vi "BlueM_Excel-gain.vi"() -> ()   [LabVIEW 2018]
panel:
  out "PID gain schedule":T1(array[cluster])=[{"PID gains"={"proportional gain (Kc)"=1.0, "integral time (Ti, min)"=0.01, "derivative time (Td, min)"=0.0}, "max value"=100.0}] {"max value" format="%.2f"; "PID gains"."derivative time (Td, min)" format="%.3f"; "PID gains"."integral time (Ti, min)" format="%.3f"; "PID gains"."proportional gain (Kc)" format="%.3f"}
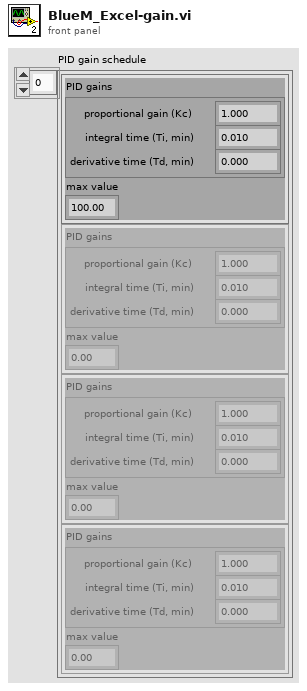
[diagram p1: front panel]
types:
  T1 = cluster{"PID gains":cluster{"proportional gain (Kc)":dbl, "integral time (Ti, min)":dbl, "derivative time (Td, min)":dbl}, "max value":dbl}[]
  T2 = enum16{"open", "replace", "create", "open or create", "replace or create", "replace or create with confirmation"}
  T3 = cluster{"[0]":dbl, "[1]":dbl, "[2]":dbl, "[3]":dbl, "[4]":dbl, "[5]":dbl, "[6]":dbl, "[7]":dbl, "[8]":dbl}
  T4 = cluster{cluster{"[1]":dbl, "[2]":dbl, "[3]":dbl}, "[0]":dbl}
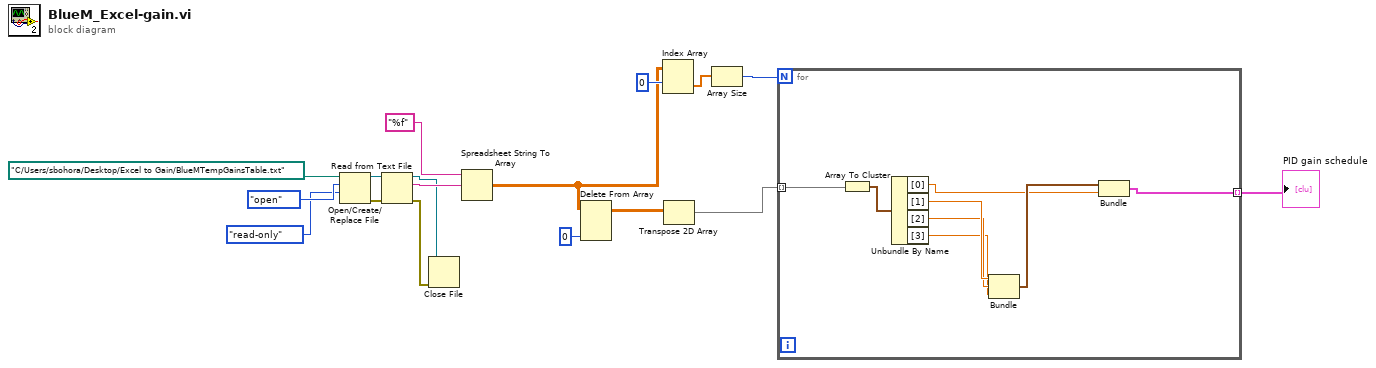
[diagram p0: block diagram]
diagram:
  n1 = Open/Create/Replace File(file path (use dialog)=path "C:/Users/sbohora/Desktop/Excel to Gain/BlueMTempGainsTable.txt", operation (0:open)=T2."open", access (0:read/write)=enum16{"read/write", "read-only", "write-only"}."read-only") -> (refnum out=w15:refnum<file>, error out=w16:errorcluster)  [unwired: 3 in, 1 out]
  n2 = Read from Text File(file (use dialog)=w15, error in=w16) -> (refnum out=w12:refnum<file>, text=w14:string, error out=w11:errorcluster)  [unwired: 2 in, 1 out]
  n3 = Close File(refnum=w12, error in=w11) -> ()  [unwired: 2 out]
  n4 = Spreadsheet String To Array(format string="%f", spreadsheet string=w14) -> (array=w2:dbl[][])  [unwired: 2 in]
  n5 = Delete From Array(array=w2, index (col)=0 ("disabled index (col)")) -> (array with subset deleted=w3:dbl[][])  [unwired: 2 in, 1 out]
  n6 = Index Array(array=w2, index (row)=0) -> (element=w7:dbl[])  [unwired: 1 in]
  n7 = Transpose 2D Array(2D array=w3) -> (transposed array=w5:dbl[][])
  n8 = Array Size(array=w7) -> (size(s)=w8:i32)
  n9 = for {
    N: w8 -> [_]
    tunnel: w5 -> [w24] mode=indexing
    tunnel: [w25] -> w4 mode=indexing
    n10 = Array To Cluster(array=w24) -> (cluster=w23:T3)
    n11 = Unbundle By Name(w23) -> ("[0]"=w18:dbl, "[1]"=w22:dbl, "[2]"=w21:dbl, "[3]"=w20:dbl)
    n12 = Bundle("[1]"=w22, "[2]"=w21, "[3]"=w20) -> (w19:cluster{"[1]":dbl, "[2]":dbl, "[3]":dbl})  [unwired: 1 in]
    n13 = Bundle(w19, "[0]"=w18) -> (w25:T4)  [unwired: 1 in]
  }
  "PID gain schedule" <- w4
